vi "pop-up debug.vi"() -> ()   [LabVIEW 2020]
uses:
  Type Defs/Motor Pop-up Config Type Def.ctl
  Type Defs/Motors Type Def.ctl
  Type Defs/Motor Type Type Def.ctl
  Type Defs/Pop-up Corner Type Def.ctl
  <vilib>/Utility/miscctls.llb/LVPositionTypeDef.ctl
panel:
  out "Motor_Sel":bool=TRUE
  in  "Motor Descriptions":string[](array[string])=["Wet Silo\nDrag", "Wet Bin\nDrag", "Wet Silo\nFan", "Wet Bin\nFan", "Dryer\nDrag", "Dryer\nFan", "Dry Bin\nFan", "Dry Bin\nDrag", "Dry Bin\nTop Feed", "U-Trough", "Leg"]
  in  "VFD Pop-up":enum32{"Page 1"}(tab)
  in  "Speed -100":bool
  in  "Speed -10":bool
  in  "Speed +10":bool
  in  "Speed +100":bool
  out "VFD_Fault":bool=TRUE caption="Fault"
  out "VFD_Running":bool=TRUE caption="Running"
  in  "VFD_Toggle":bool
  out "Motor_Speed":u16=140 caption="bu"
  in  "Motor Pop-up":enum32{"Page 1"}(tab)
  out "Motor_Overload":bool=TRUE caption="Overload"
  out "Motor_Running":bool=TRUE caption="Running"
  in  "Motor_Toggle":bool
  out "DB_Fan":bool=TRUE
  in  "Motor Pop-ups":T1[](array[typedef])=[{"Motor"=enum."WS_Drag", "Motor Type"=enum."MS", "Pop-up Corner"=enum."Top Right"}]
  # "rpm"
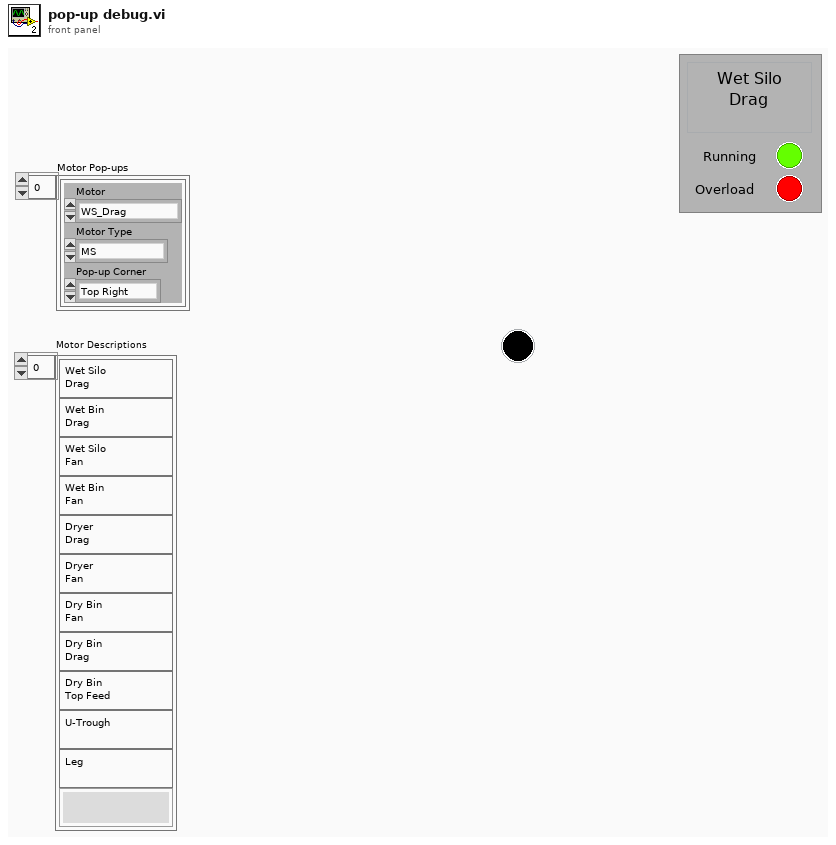
[diagram p1: front panel]
types:
  T1 = typedef "Motor Pop-up Config Type Def.ctl" = cluster{"Motor":T2, "Motor Type":T3, "Pop-up Corner":T4}
  T2 = typedef "Motors Type Def.ctl" = enum16{"WS_Drag", "WB_Drag", "WS_Fan", "WB_Fan", "Dryer_Drag", "Dryer_Fan", "DB_Fan", "DB_Drag", "DB_Top_Feed", "U-Trough", "Leg"}
  T3 = typedef "Motor Type Type Def.ctl" = enum16{"MS", "VFD"}
  T4 = typedef "Pop-up Corner Type Def.ctl" = enum16{"Top Left", "Top Right", "Bottom Left", "Bottom Right"}
  T5 = typedef "LVPositionTypeDef.ctl" = cluster{"Left":i32, "Top":i32}
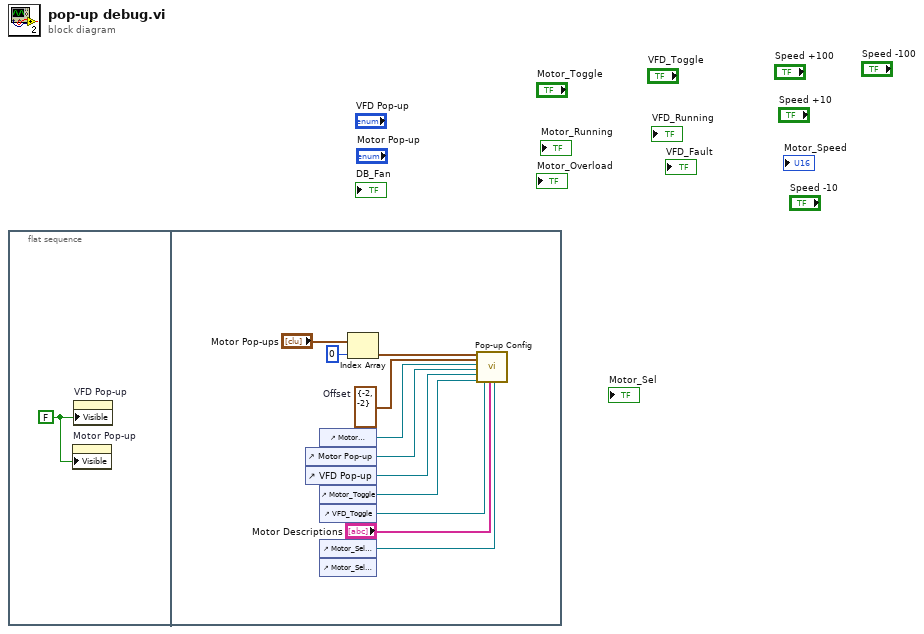
[diagram p0: block diagram]
diagram:
  n1 = flat-sequence {
    frame #0 {
      w1 = FALSE ("Visible")
      n2 = property on="Motor Pop-up" class="TabCtl (strict)"("Visible"=w1) -> ()  [unwired: 2 in, 2 out]
      n3 = property on="VFD Pop-up" class="TabCtl (strict)"("Visible"=w1) -> ()  [unwired: 2 in, 2 out]
    }
    frame #1 {
      w9 = T5 {"Left"=-2, "Top"=-2}  # Offset
      n4 = control-ref of="Motor Pop-up"() -> (w7:refnum<vi>)
      n5 = control-ref of="VFD Pop-up"() -> (w6:refnum<vi>)
      n6 = control-ref of="Motor Indicator"() -> (w8:refnum<vi>)
      n7 = control-ref of="Motor_Toggle"() -> (w5:refnum<vi>)
      n8 = control-ref of="VFD_Toggle"() -> (w4:refnum<vi>)
      n9 = control-ref of="Motor_Sel (Round)"() -> (w2:refnum<vi>)
      n10 = control-ref of="Motor_Sel (Square)"() -> ()  [unwired: 1 out]
      n11 = Index Array(array="Motor Pop-ups", index=0) -> (element=w10:T1)
      n12 = call "Pop-up Config.vi"("Motor Pop-up Config"=w10, "Offset"=w9, "Motor Indicator"=w8, "Motor Pop-up"=w7, "VFD Pop-up"=w6, "Motor_Toggle"=w5, "VFD_Toggle"=w4, "Motor Descriptions"="Motor Descriptions", "Motor_Sel (Round)"=w2) -> ()  [unwired: 11 in]
    }
  }
